vi "Handle Last Ack Core.vi"(4 "error in":errorcluster, 6 "Last Ack":refnum<class "Last Ack.lvclass">, 7 "UI Actor in":refnum<class "UI Actor.lvclass">) -> (0 "error out":errorcluster, 3 "UI Actor out":refnum<class "UI Actor.lvclass">)   [LabVIEW 2014, in "Device Test.lvlib" / "UI Actor.lvclass"]
doc: "(<B>Filename</B>: Actor Framework.lvlib:Actor.lvclass:Handle Last Ack Core.vi)\n\nDefines how the caller actor responds to the Last Ack message from a nested actor. The Last Ack message is the final message a nested actor sends to its caller before it shuts down. The message contains information about the final state of the nested actor.\n\nBy default, this method does nothing except return any error the nested actor sent. A descendant class may override this method to define behavior."
uses:
  UI Actor.lvclass
  <vilib>/ActorFramework/LastAck/Last Ack.lvclass
  UI Actor.lvclass/UI Actor.ctl
  <vilib>/ActorFramework/Actor/Actor.lvclass/Actor.ctl
  <vilib>/ActorFramework/Message Enqueuer/Message Enqueuer.lvclass/Message Enqueuer.ctl
  <vilib>/ActorFramework/Message Enqueuer/Init from Existing Queue.vi
  <vilib>/ActorFramework/Message Enqueuer/Enqueue.vi
  <vilib>/ActorFramework/Message Priority Queue/Priority Enqueue.vi
  <vilib>/ActorFramework/Message Enqueuer/Message Enqueuer.lvclass
  <vilib>/ActorFramework/Stop Msg/Stop Msg.lvclass
  <vilib>/ActorFramework/Actor/Actor.lvclass
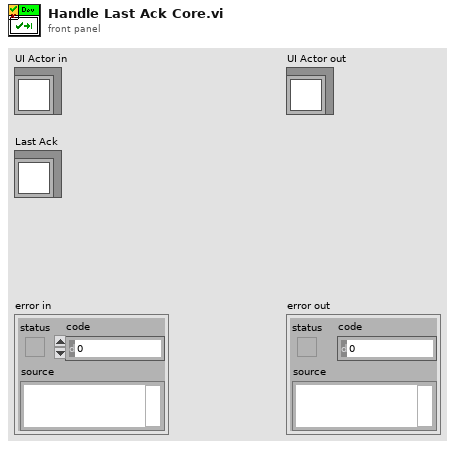
[diagram p1: front panel]
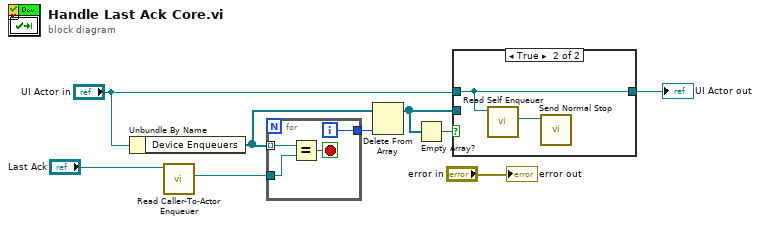
[diagram p0: block diagram]
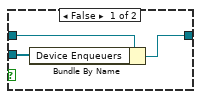
[diagram p2: hidden frame]
diagram:
  n1 = Unbundle By Name("UI Actor in") -> ("Device Enqueuers"=w6:refnum<class "Message Enqueuer.lvclass">[])
  n2 = call <vilib>:"Read Caller-To-Actor Enqueuer.vi"("Last Ack"="Last Ack") -> ("Caller-to-Actor Enqueuer"=w7:refnum<class "Message Enqueuer.lvclass">)  [unwired: 10 in]
  n3 = for {
    tunnel: w6 -> [w13] mode=indexing
    tunnel: w7 -> [w12]
    tunnel: [w10] -> w5
    i -> [w10]
    stop <- w11 stop-if-true
    n4 = Equal?(x=w13, y=w12) -> (x = y?=w11:bool)
  }
  n5 = Delete From Array(array=w6, index=w5) -> (array with subset deleted=w4:refnum<class "Message Enqueuer.lvclass">[])  [unwired: 1 in, 1 out]
  n6 = Empty Array?(array=w4) -> (empty?=w1:bool)
  n7 = case shown="True" w1 {
    tunnel: w4 -> [w16 _]
    tunnel: [w15 w18] -> w3
    tunnel: "UI Actor in" -> [w14 w18]
    frame False {
      n8 = Bundle By Name(cluster=w14, "Device Enqueuers"=w16) -> (w15:refnum<class "UI Actor.lvclass">)
    }
    frame True {
      n9 = call <vilib>:"Read Self Enqueuer.vi"("Actor"=w18) -> ("Self Enqueuer"=w17:refnum<class "Message Enqueuer.lvclass">)  [unwired: 10 in]
      n10 = call <vilib>:"Send Normal Stop.vi"("Message Enqueuer"=w17) -> ()  [unwired: 10 in, 1 out]
    }
  }
  "UI Actor out" <- w3
  "error out" <- "error in"
